vi "Get Indicator.vi"(8 "error in (no error)":errorcluster, 11 "Panel_UI in":refnum<class "Panel_UI.lvclass">) -> (0 "error out":errorcluster, 2 "Indicater":i32, 3 "Panel_UI out":refnum<class "Panel_UI.lvclass">)   [LabVIEW 2015, in "Panel_UI.lvclass"]
uses:
  Panel_UI.lvclass
  Panel_UI.lvclass/Panel_UI.ctl
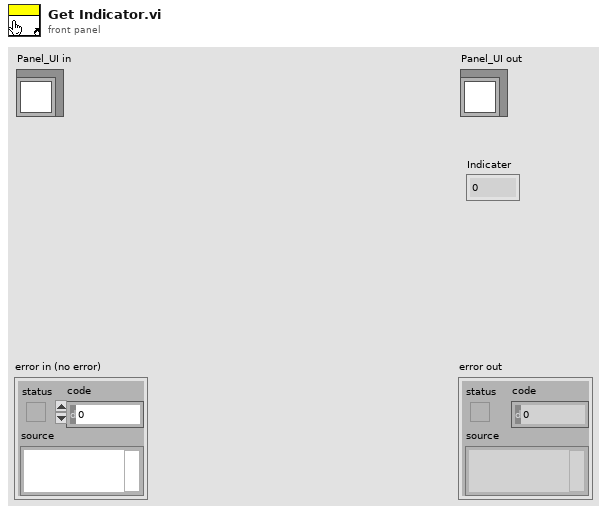
[diagram p1: front panel]
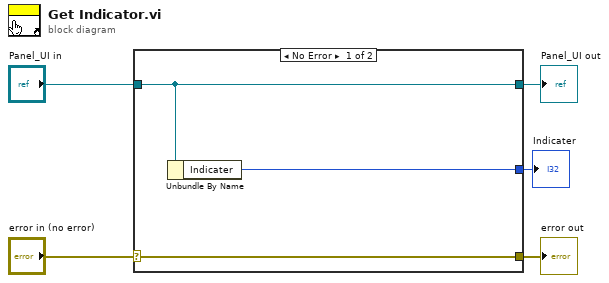
[diagram p0: block diagram]
diagram:
  n1 = case shown="No Error" "error in (no error)" {
    selector: "error in (no error)" -> [w8 w9]
    tunnel: [w8 w9] -> w4
    tunnel: [w7 w10] -> w2
    tunnel: "Panel_UI in" -> [w7 w10]
    tunnel: [w6 _] -> w1
    frame No Error {
      n2 = Unbundle By Name(w7) -> ("Indicater"=w6:i32)
    }
    frame Error {
    }
  }
  "error out" <- w4
  "Panel_UI out" <- w2
  "Indicater" <- w1
